vi "Set_Keystate_String_for_HP4275A.vi"(0 "Display A":u16(ring) items=["A1", "A2", "A3", "A4"], 1 "Display B":u16(ring) items=["B1", "B2", "B3", "B1,B3", "B2", "B1,B2,B3"], 2 "Circuit Mode":u16(ring) items=["C1", "C2", "C3"], 3 "Dev Measure":u16(ring) items=["D0", "D1", "D2"], 4 "Freq. Step":u16(ring) items=["F11", "F12", "F13", "F14", "F15", "F16", "F17", "F18", "F19", "F20", "F21", "F22"], 5 "High Resolution Mode":u16(ring) items=["H0", "H1"], 6 "Data Ready":u16(ring) items=["I0", "I1"], 7 "error in":errorcluster, 8 "Key State Out":u16(ring) items=["K", ""], 9 "Reference Value":u16(ring) items=["ST", "RE"], 10 "Multiplier":u16(ring) items=["M1", "M2", "M3"], 12 "Trigger":u16(ring) items=["T1", "T2"], 13 "Execute":u16(ring) items=["T1", "T2"]) -> (27 "error out":errorcluster)   [LabVIEW 2020]
panel:
  # "Data Ready\nOff -I0\nOn - I1"
  # "Display A\nCapacitance or Gate Resistance Test\nA2(Cap) or A3(Rg)"
  # "Key State Out\nK\n<blank>"
  # "Display B\nD - Dissipation Factor\nQ - Quality Factor\nESR/G - Equivalent series R or G\nX/B - Reactance/Susceptance L or C in R measurements\nL/C - Inductance/Capacitance\nTheta - Phase angle in Z measurements"
  # "Multiplier\nX0.01 - M1\nX0.1 - M2\nX1 - M3"
  # "Circuit Mode\nAuto - C1\nSeries - C2\nParallel - C3"
  # "Reference Value\nStore - ST\nRecall - RE"
  # "Deviation Measurement\nOff - D0\nDelta - D1\nDelta % - D2"
  # "Trigger\nInternal - T1\nExternal - T2"
  # "Frequency Step\n10 kHz - F11                     1 MHz - F17\n20(30) kHz - F12              2(3) MHz - F18\n40(50) kHz - F13              4(5) MHz - F19\n100 kHz - F14                   10 MHz - F20\n200(300) kHz - F15           *1 - F21\n400(500) kHz - F16           *2 - F22"
  # "Execute\nExecute command - E\nNo execution - \"\" (blank)"
  # "High Resolution Mode\nOff - H0\nOn - H1"
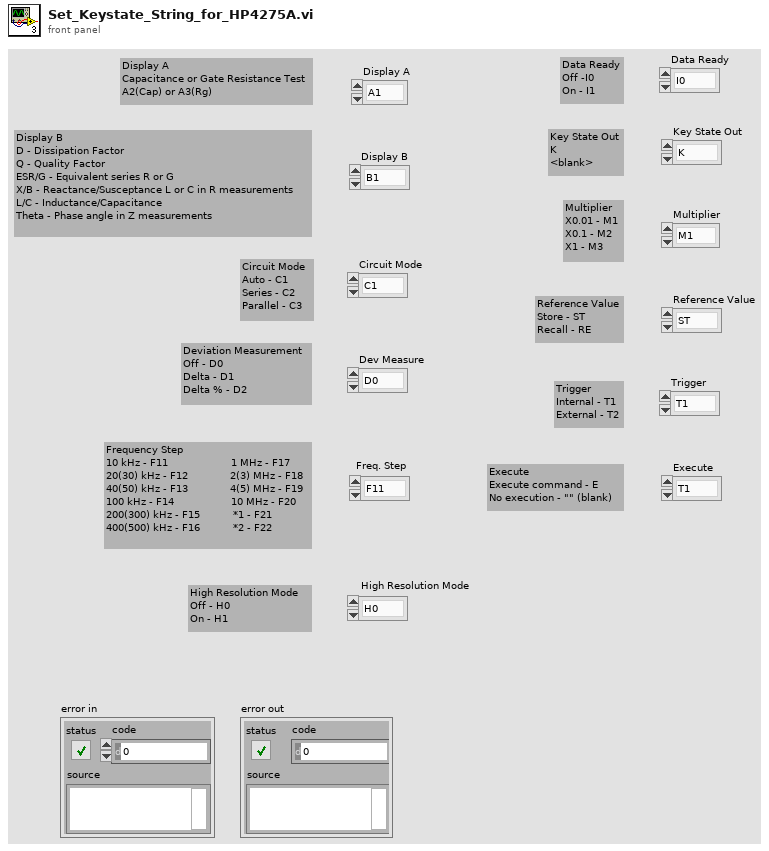
[diagram p1: front panel]
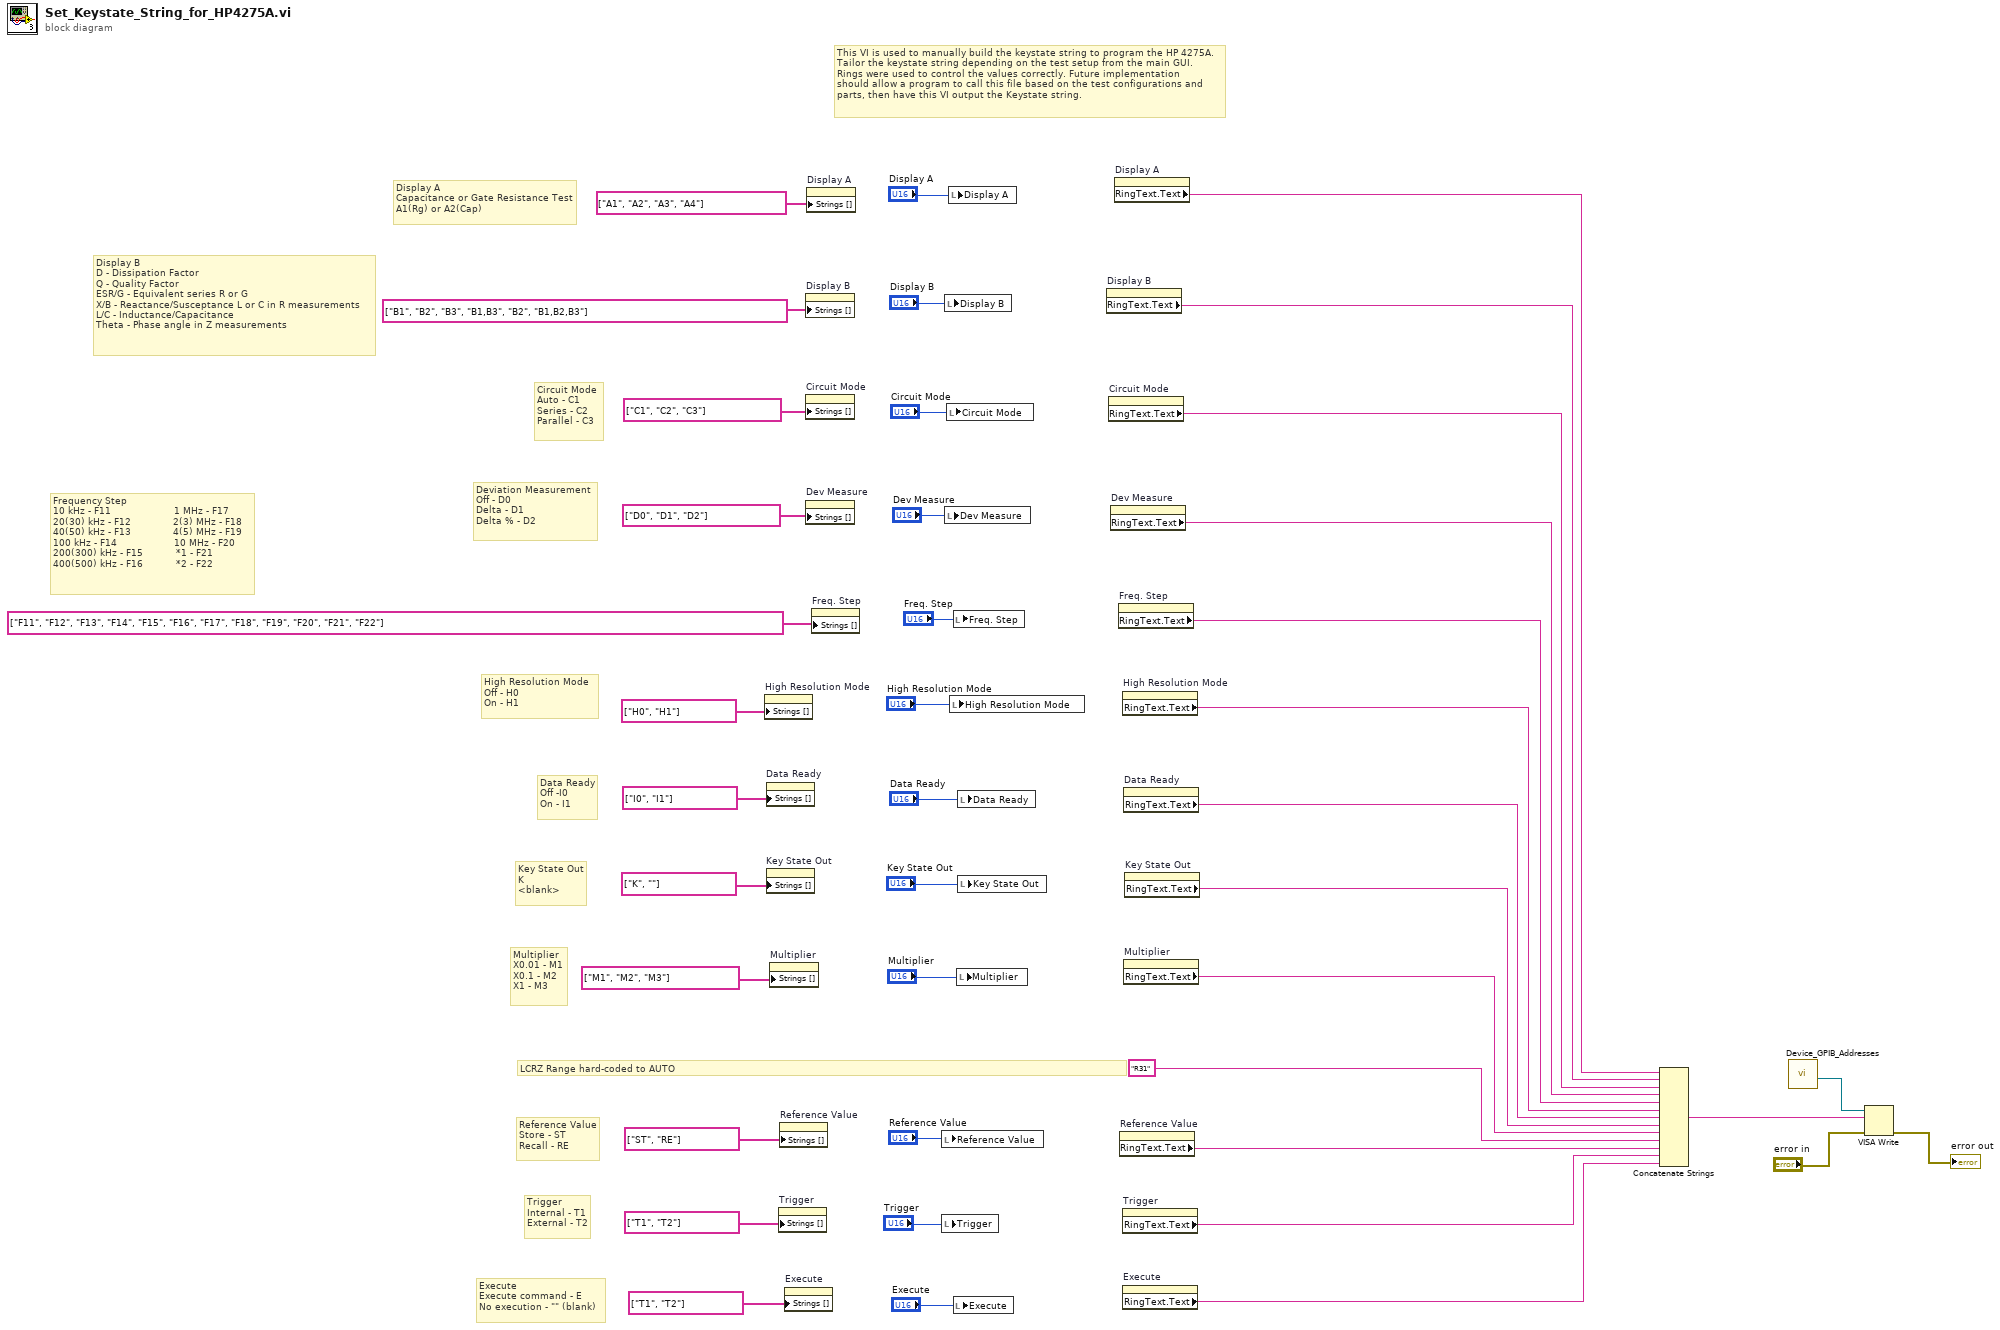
[diagram p0: block diagram]
diagram:
  # "This VI is used to manually build the keystate string to program the HP 4275A.\nTailor the keystate string depending on the test setup from the main GUI.\nRings were used to control the values correctly. Future implementation\nshould allow a program to call this file based on the test configurations and\nparts, then have this VI output the Keystate string."
  # "Multiplier\nX0.01 - M1\nX0.1 - M2\nX1 - M3"
  # "Execute\nExecute command - E\nNo execution - \"\" (blank)"
  # "Trigger\nInternal - T1\nExternal - T2"
  # "Reference Value\nStore - ST\nRecall - RE"
  # "LCRZ Range hard-coded to AUTO"
  # "Key State Out\nK\n<blank>"
  # "Data Ready\nOff -I0\nOn - I1"
  # "High Resolution Mode\nOff - H0\nOn - H1"
  # "Frequency Step\n10 kHz - F11                     1 MHz - F17\n20(30) kHz - F12              2(3) MHz - F18\n40(50) kHz - F13              4(5) MHz - F19\n100 kHz - F14                   10 MHz - F20\n200(300) kHz - F15           *1 - F21\n400(500) kHz - F16           *2 - F22"
  # "Deviation Measurement\nOff - D0\nDelta - D1\nDelta % - D2"
  # "Circuit Mode\nAuto - C1\nSeries - C2\nParallel - C3"
  # "Display B\nD - Dissipation Factor\nQ - Quality Factor\nESR/G - Equivalent series R or G\nX/B - Reactance/Susceptance L or C in R measurements\nL/C - Inductance/Capacitance\nTheta - Phase angle in Z measurements"
  # "Display A\nCapacitance or Gate Resistance Test\nA1(Rg) or A2(Cap)"
  n1 = property on="High Resolution Mode" class="Ring (strict)"("Strings []"=string[] ["H0", "H1"]) -> ()  [unwired: 2 in, 2 out]
  n2 = property on="Data Ready" class="Ring (strict)"("Strings []"=string[] ["I0", "I1"]) -> ()  [unwired: 2 in, 2 out]
  n3 = property on="Key State Out" class="Ring (strict)"("Strings []"=string[] ["K", ""]) -> ()  [unwired: 2 in, 2 out]
  n4 = property on="Multiplier" class="Ring (strict)"("Strings []"=string[] ["M1", "M2", "M3"]) -> ()  [unwired: 2 in, 2 out]
  n5 = property on="Trigger" class="Ring (strict)"("Strings []"=string[] ["T1", "T2"]) -> ()  [unwired: 2 in, 2 out]
  n6 = property on="Reference Value" class="Ring (strict)"("Strings []"=string[] ["ST", "RE"]) -> ()  [unwired: 2 in, 2 out]
  n7 = property on="Execute" class="Ring (strict)"("Strings []"=string[] ["T1", "T2"]) -> ()  [unwired: 2 in, 2 out]
  n8 = property on="Display B" class="Ring (strict)"("Strings []"=string[] ["B1", "B2", "B3", "B1,B3", "B2", "B1,B2,B3"]) -> ()  [unwired: 2 in, 2 out]
  n9 = property on="Circuit Mode" class="Ring (strict)"("Strings []"=string[] ["C1", "C2", "C3"]) -> ()  [unwired: 2 in, 2 out]
  n10 = property on="Dev Measure" class="Ring (strict)"("Strings []"=string[] ["D0", "D1", "D2"]) -> ()  [unwired: 2 in, 2 out]
  n11 = property on="Display A" class="Ring (strict)"("Strings []"=string[] ["A1", "A2", "A3", "A4"]) -> ()  [unwired: 2 in, 2 out]
  n12 = property on="Freq. Step" class="Ring (strict)"("Strings []"=string[] ["F11", "F12", "F13", "F14", "F15", "F16", "F17", "F18", "F19", "F20", "F21", "F22"]) -> ()  [unwired: 2 in, 2 out]
  n13 = local write "Reference Value"("Reference Value") -> ()
  n14 = local write "Trigger"("Trigger") -> ()
  n15 = local write "Display B"("Display B") -> ()
  n16 = local write "Dev Measure"("Dev Measure") -> ()
  n17 = local write "Circuit Mode"("Circuit Mode") -> ()
  n18 = local write "Display A"("Display A") -> ()
  n19 = local write "High Resolution Mode"("High Resolution Mode") -> ()
  n20 = local write "Freq. Step"("Freq. Step") -> ()
  n21 = local write "Execute"("Execute") -> ()
  n22 = local write "Multiplier"("Multiplier") -> ()
  n23 = local write "Data Ready"("Data Ready") -> ()
  n24 = local write "Key State Out"("Key State Out") -> ()
  n25 = property on="Display B" class="Ring (strict)"() -> ("RingText.Text"=w21:string)  [unwired: 2 in, 2 out]
  n26 = property on="Circuit Mode" class="Ring (strict)"() -> ("RingText.Text"=w19:string)  [unwired: 2 in, 2 out]
  n27 = property on="Dev Measure" class="Ring (strict)"() -> ("RingText.Text"=w17:string)  [unwired: 2 in, 2 out]
  n28 = property on="Display A" class="Ring (strict)"() -> ("RingText.Text"=w23:string)  [unwired: 2 in, 2 out]
  n29 = property on="Freq. Step" class="Ring (strict)"() -> ("RingText.Text"=w15:string)  [unwired: 2 in, 2 out]
  n30 = property on="Reference Value" class="Ring (strict)"() -> ("RingText.Text"=w5:string)  [unwired: 2 in, 2 out]
  n31 = property on="High Resolution Mode" class="Ring (strict)"() -> ("RingText.Text"=w13:string)  [unwired: 2 in, 2 out]
  n32 = property on="Trigger" class="Ring (strict)"() -> ("RingText.Text"=w3:string)  [unwired: 2 in, 2 out]
  n33 = property on="Execute" class="Ring (strict)"() -> ("RingText.Text"=w1:string)  [unwired: 2 in, 2 out]
  n34 = property on="Data Ready" class="Ring (strict)"() -> ("RingText.Text"=w11:string)  [unwired: 2 in, 2 out]
  n35 = property on="Multiplier" class="Ring (strict)"() -> ("RingText.Text"=w7:string)  [unwired: 2 in, 2 out]
  n36 = property on="Key State Out" class="Ring (strict)"() -> ("RingText.Text"=w9:string)  [unwired: 2 in, 2 out]
  n37 = Concatenate Strings(w23, w21, w19, w17, w15, w13, w11, w9, w7, "R31", w5, w3, w1) -> (w37:string)
  n38 = call "Device_GPIB_Addresses.vi"() -> ("HP 4275A Address"=w41:refnum<visa-resource-name>)  [unwired: 9 in, 2 out]
  n39 = VISA Write(VISA resource name=w41, write buffer=w37, error in (no error)="error in") -> (error out=→"error out":errorcluster)  [unwired: 2 out]
